vi "CAN Control Timming.vi"() -> ()   [LabVIEW 2010]
uses:
  <vilib>/Platform/storage/lvStorage.llb/xStorage/Open Data Storage/Open Data Storage.xnode
  <vilib>/Platform/storage/lvStorage.llb/_openFunction.ctl
  <vilib>/Platform/storage/lvStorage.llb/xStorage/Set Properties/Set Properties.xnode
  <vilib>/Platform/storage/lvStorage.llb/xStorage/Write Data/Write Data.xnode
  <vilib>/Platform/storage/Storage.llb/usiOverwriteOptions.ctl
  <vilib>/Platform/storage/Storage.llb/usiSequenceRepresentation.ctl
  <vilib>/Platform/storage/lvStorage.llb/xStorage/Close Data Storage/Close Data Storage.xnode
  <instrlib>/Tektronix DPO MSO 2000 4000 Series/Public/Data/Read (Single Waveform).vi
  <instrlib>/Tektronix DPO MSO 2000 4000 Series/Public/Data/Read (Multiple Waveforms).vi
  <vilib>/Platform/storage/lvStorage.llb/_openStorageWithRootAutoDetect.vi
  <vilib>/Platform/storage/lvStorage.llb/xStorage/xStorageSupp/ErrorOut.vi
  <vilib>/Platform/storage/Storage.llb/__savePropString.vi
  <vilib>/Platform/storage/Storage.llb/__savePropTime.vi
  <vilib>/Platform/storage/Storage.llb/_createExplicitChildObject.vi
  <vilib>/Platform/storage/lvStorage.llb/_prepDDT.vi
  <vilib>/Platform/storage/lvStorage.llb/_getChannelNameFromDDT.vi
  <vilib>/Platform/storage/lvStorage.llb/_saveDDT.vi
  <vilib>/Platform/storage/Storage.llb/Get Object Info.vi
  <vilib>/Platform/storage/Storage.llb/__closeStorageFromObject.vi
  <instrlib>/Tektronix DPO MSO 2000 4000 Series/Tektronix DPO MSO 2000 4000 Series.lvlib
panel:
  out "error out":errorcluster
  in  "Error Range":dbl min=0.0 max=5.0 step=0.1 format="%#.3g"
  in  "DPO-4034 IP Adress":string
  in  "Port":u16(ring) items=["AMB 1", "AMB 2", "AMB 3", "AMB 4", "AMB 5", "AMB 18"]
  in  "ABM-S/N":string
  in  "Assembled by":string="Alexis Ibarra"
  in  "Tab Control":enum32{"Diferential"}(tab)
  out "TIMB":waveform(dbl)(graph)
  out "CAN Diferential":waveform(dbl)(graph)
  in  "Maximum Time (10000ms)":u32=20000
  in  "Channel B (1: Channel 2)":u16(ring)=1 items=["Channel 1", "Channel 2", "Channel 3", "Channel 4", "Math", "Reference 1", "Reference 2", "Reference 3", "Reference 4"]
  in  "Channel A (0: Channel 1)":u16(ring) items=["Channel 1", "Channel 2", "Channel 3", "Channel 4", "Math", "Reference 1", "Reference 2", "Reference 3", "Reference 4"]
  out "UP":dbl
  out "DOWN":dbl
  out "?":bool
  out "?":bool
  out "STATUS":string
  out "Delay":dbl format="%^#_6g"
  out "average":dbl
  out "CAN+TIMB":waveform(dbl)[](graph)
  # "TCPIP0::10.195.18.178::inst0::INSTR"
  # "Actually ip address\n10.195.18.178"
  # "%"
  # "Error Limit"
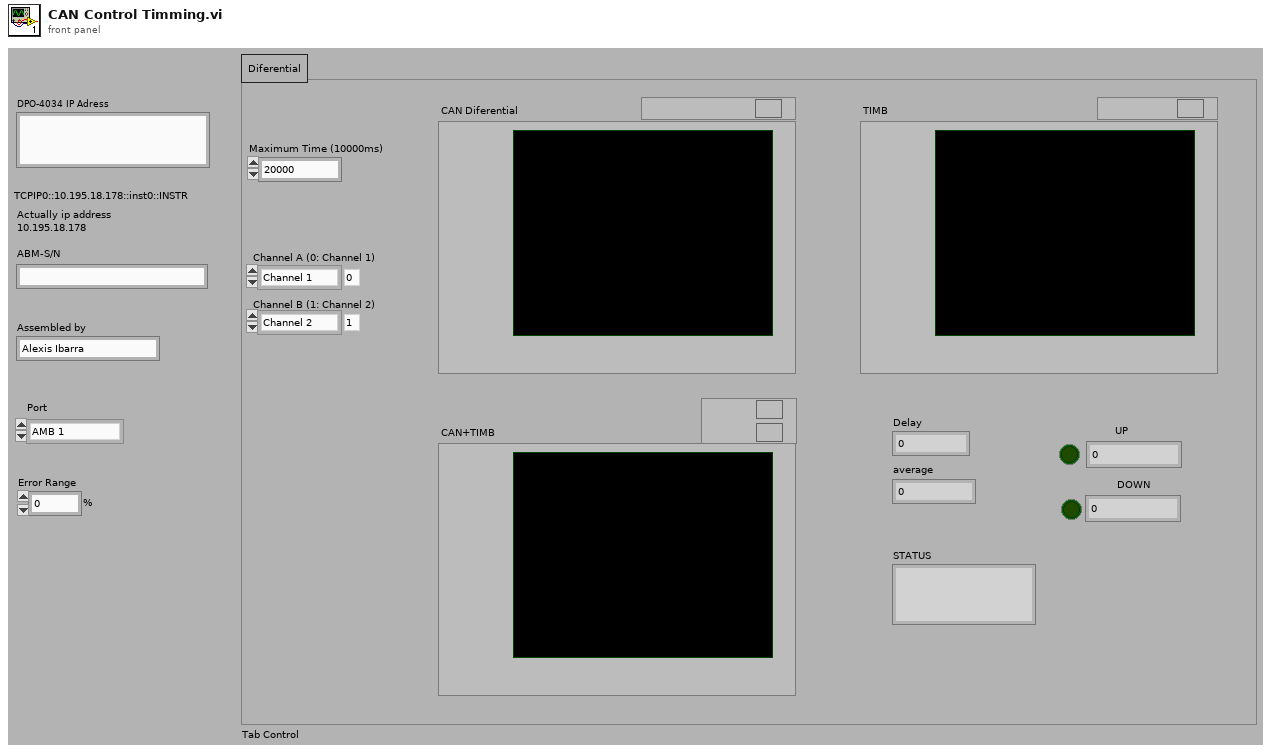
[diagram p1: front panel]
types:
  T1 = enum16{"UPDATE", "READ", "QUERY", "CREATE CHILD", "CREATE", "CONNECT", "DISCONNECT"}
  T2 = typedef "usiOverwriteOptions.ctl" = enum16{"Append values", "Replace values at index", "Replace all values", "Append if timeline aligns"}
  T3 = typedef "usiSequenceRepresentation.ctl" = enum16{"explicit", "implicit"}
  T4 = typedef "_openFunction.ctl" = enum16{"open", "open or create", "create or replace", "create", "open (read only)"}
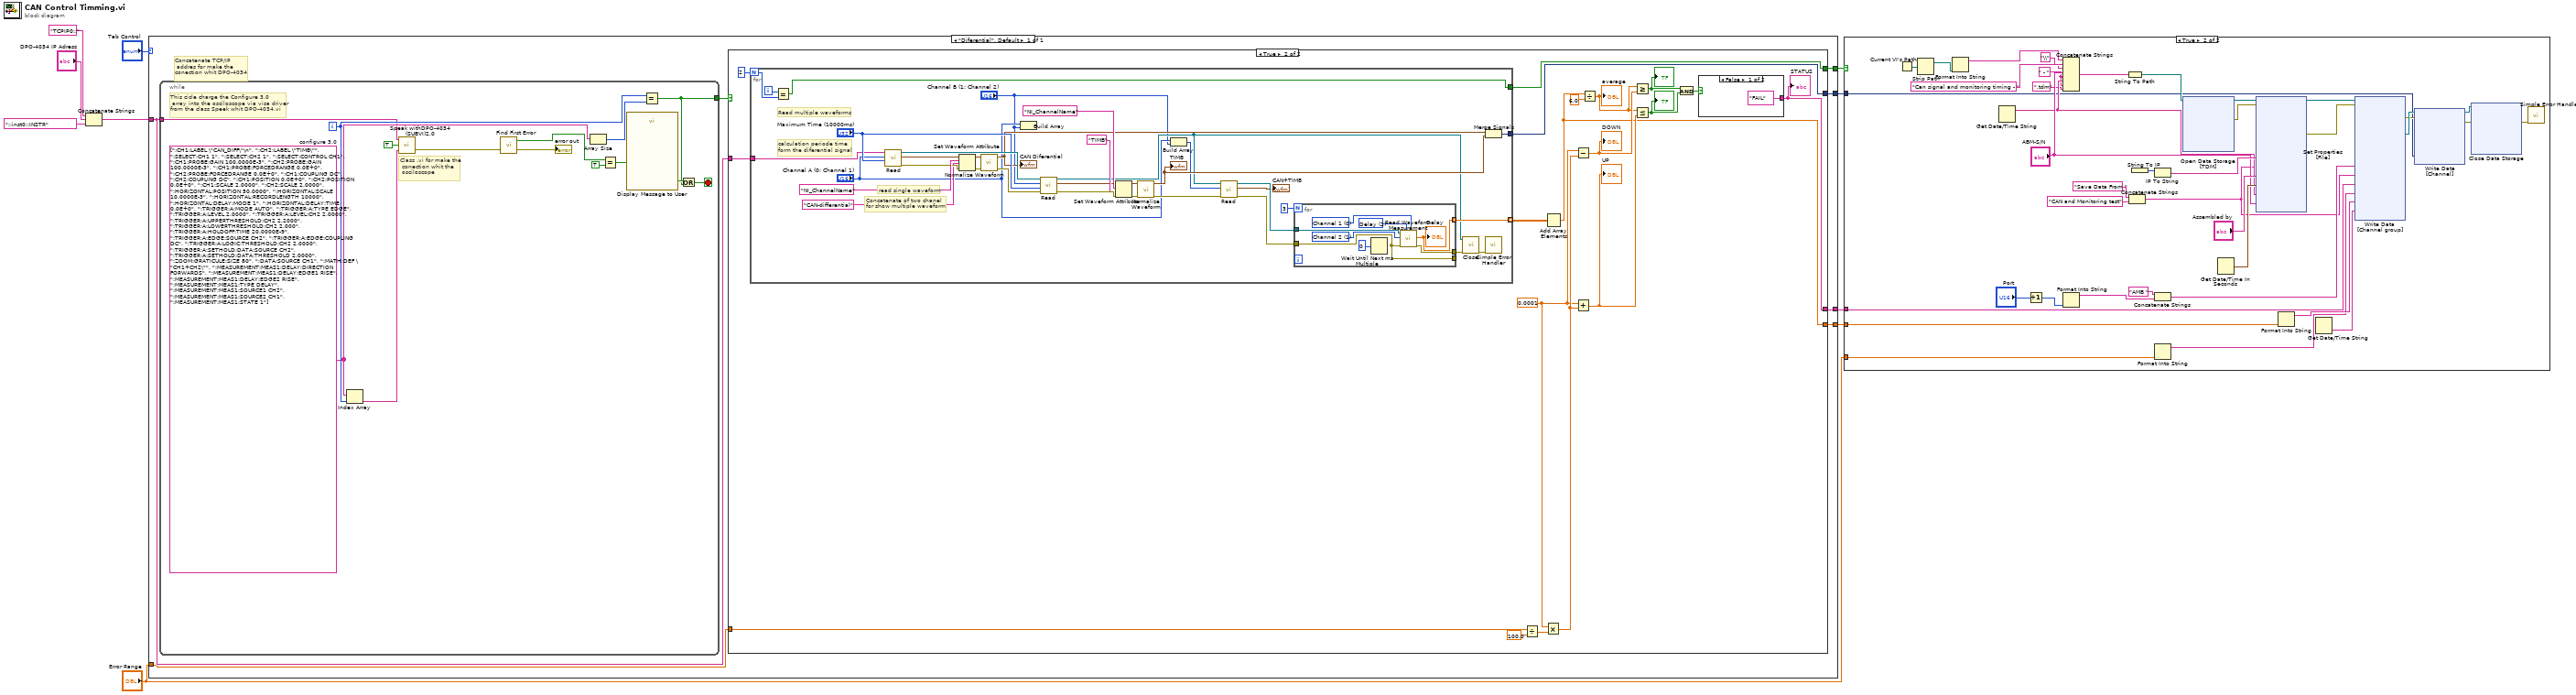
[diagram p0: block diagram]
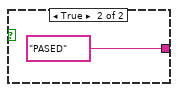
[diagram p4: hidden frame]
diagram:
  n1 = Concatenate Strings("TCPIP0::", "DPO-4034 IP Adress", "::inst0::INSTR") -> (w4:string)
  n2 = case shown="\"Diferential\", Default" "Tab Control" {
    tunnel: [w16] -> w9
    tunnel: [w15] -> w8
    tunnel: w4 -> [w14]
    tunnel: [w13] -> w3
    tunnel: "Error Range" -> [w12]
    tunnel: [w11] -> w1
    frame "Diferential", Default {
      # "Concatenate TCP/IP\n addres for make the \nconection whit DPO-4034"
      n3 = while {
        tunnel: w14 -> [w84]
        tunnel: [w81] -> w17
        i -> [w93]
        stop <- w82 stop-if-true
        w88 = string[] [":CH1:LABEL \"CAN_DIFF\"\n", ":CH2:LABEL \"TIMB\"", ":SELECT:CH1 1", ":SELECT:CH2 1", ":SELECT:CONTROL CH1", ":CH1:PROBE:GAIN 100.0000E-3", ":CH2:PROBE:GAIN 100.0000E-3", ":CH1:PROBE:FORCEDRANGE 0.0E+0", ":CH2:PROBE:FORCEDRANGE 0.0E+0", ":CH1:COUPLING DC", ":CH2:COUPLING DC", ":CH1:POSITION 0.0E+0", ":CH2:POSITION 0.0E+0", ":CH1:SCALE 2.0000", ":CH2:SCALE 2.0000", ":HORIZONTAL:POSITION 50.0000", ":HORIZONTAL:SCALE 10.0000E-3", ":HORIZONTAL:RECORDLENGTH 10000", ":HORIZONTAL:DELAY:MODE 1", ":HORIZONTAL:DELAY:TIME 0.0E+0", ":TRIGGER:A:MODE AUTO", ":TRIGGER:A:TYPE EDGE", ":TRIGGER:A:LEVEL 2.0000", ":TRIGGER:A:LEVEL:CH2 2.0000", ":TRIGGER:A:UPPERTHRESHOLD:CH2 2.2000", ":TRIGGER:A:LOWERTHRESHOLD:CH2 2.000", ":TRIGGER:A:HOLDOFF:TIME 20.0000E-9", ":TRIGGER:A:EDGE:SOURCE CH2", ":TRIGGER:A:EDGE:COUPLING DC", ":TRIGGER:A:LOGIC:THRESHOLD:CH2 2.0000", ":TRIGGER:A:SETHOLD:DATA:SOURCE CH2", ":TRIGGER:A:SETHOLD:DATA:THRESHOLD 2.0000", ":ZOOM:GRATICULE:SIZE 80", ":DATA:SOURCE CH1", ":MATH:DEF \"CH1+CH2\"", ":MEASUREMENT:MEAS1:DELAY:DIRECTION FORWARDS", ":MEASUREMENT:MEAS1:DELAY:EDGE1 RISE", ":MEASUREMENT:MEAS1:DELAY:EDGE2 RISE", ":MEASUREMENT:MEAS1:TYPE DELAY", ":MEASUREMENT:MEAS1:SOURCE1 CH2", ":MEASUREMENT:MEAS1:SOURCE2 CH1", ":MEASUREMENT:MEAS1:STATE 1"]  # configure 3.0
        # "Class .vi for make the\n conection whit the\n osciloscope"
        # "This cicle charge the Configure 3.0\n array into the osciloscope via visa driver \nfrom the class Speek whit DPO-4034.vi"
        n4 = Index Array "Index Array"(array=w88, index=w93) -> (element=w94:string)
        n5 = call "Speak withDPO-4034 (SUBVI)2.0.vi"("Send Command"=w94, "Send:  TRUE\nRecive: FALSE"=TRUE, "VISA Resource Name"=w84) -> ("error out"=w90:errorcluster)  [unwired: 1 out]
        n6 = call <vilib>:"Find First Error.vi"("error in (no error)"=w90) -> ("error out"=→"error out":errorcluster, "error?"=w85:bool)  [unwired: 3 in]
        n7 = Array Size(array=w88) -> (size(s)=w92:i32)
        n8 = Equal?(x=w85, y=TRUE) -> (x = y?=w87:bool)
        n9 = call "Display Message to User"("Enable"=w87) -> ("OK"=w83:bool)  [unwired: 9 in, 1 out]
        n10 = Equal?(x=w93, y=w92) -> (x = y?=w81:bool)
        n11 = Or(x=w83, y=w81) -> (x .or. y?=w82:bool)
      }
      n12 = case shown="True" w17 {
        tunnel: w14 -> [_ w36]
        tunnel: [_ w35] -> w16
        tunnel: [_ w34] -> w15
        tunnel: [_ w20] -> w13
        tunnel: w12 -> [_ w27]
        tunnel: [_ w23] -> w11
        frame False {
        }
        frame True {
          w30 = 0.0001 ("x")
          n13 = for {
            N: 2 -> [w47]
            tunnel: w36 -> [w51]
            tunnel: [w52] -> w35
            tunnel: [w46] -> w34
            tunnel: [w45] -> w18 mode=indexing
            i -> [w48]
            # "read single waveform"
            # "Concatenate of two chanel \nfor show multiple waveform"
            # "calculation periode time\nform the diferential signal"
            # "Read multiple waveforms"
            n14 = Equal?(x=w48, y=w47) -> (x = y?=w46:bool)
            n15 = call-poly <instrlib>:"Read.vi"("Maximum Time (10000ms)"="Maximum Time (10000ms)", "Channel (0: Channel 1)"="Channel A (0: Channel 1)", "VISA resource name"=w51) -> ("error out"=w67:errorcluster, "Waveform Graph"=w56:waveform(dbl), "VISA resource name out"=w69:refnum<visa-resource-name>)  [unwired: 6 in]
            n16 = Set Waveform Attribute(4:w67, 5:"CAN-differential" ("name"), 6:"NI_ChannelName" ("name"), 7:w56) -> (0:w59:errorcluster, 3:w61:waveform(dbl))  [unwired: 1 out]
            n17 = call <vilib>:"Normalize Waveform.vi"("error in (no error)"=w59, "waveform in"=w61) -> ("error out"=w58:errorcluster, "normalized waveform"=w54:waveform(dbl))  [unwired: 6 in, 2 out]
            "CAN Diferential" <- w54
            n18 = Build Array("Channel A (0: Channel 1)", "Channel B (1: Channel 2)") -> ()  [unwired: 1 out]
            n19 = call-poly <instrlib>:"Read.vi"("error in (no error)"=w58, "Maximum Time (10000ms)"="Maximum Time (10000ms)", "Channel (0: Channel 1)"="Channel B (1: Channel 2)", "VISA resource name"=w69) -> ("error out"=w64:errorcluster, "Waveform Graph"=w55:waveform(dbl), "VISA resource name out"=w42:refnum<visa-resource-name>)  [unwired: 5 in]
            n20 = Set Waveform Attribute(4:w64, 5:"TIMB" ("name"), 6:"NI_ChannelName" ("name"), 7:w55) -> (0:w57:errorcluster, 3:w60:waveform(dbl))  [unwired: 1 out]
            n21 = call <vilib>:"Normalize Waveform.vi"("error in (no error)"=w57, "waveform in"=w60) -> ("error out"=w44:errorcluster, "normalized waveform"=w53:waveform(dbl))  [unwired: 6 in, 2 out]
            "TIMB" <- w53
            n22 = Build Array("Channel A (0: Channel 1)", "Channel B (1: Channel 2)") -> (w38:u16[])
            n23 = call-poly <instrlib>:"Read.vi"("error in (no error)"=w44, "Channels"=w38, "VISA resource name"=w42) -> ("error out"=w43:errorcluster, "Waveform Data"=→"CAN+TIMB":waveform(dbl)[], "VISA resource name out"=w41:refnum<visa-resource-name>)  [unwired: 6 in]
            n24 = for {
              N: 3 -> [_]
              tunnel: w41 -> [w78]
              tunnel: [w75] -> _
              tunnel: [w76] -> w50
              tunnel: w43 -> [w75]
              tunnel: [w73] -> w45 mode=indexing
              w71 = u16 0 items=["Channel 1", "Channel 2", "Channel 3", "Channel 4", "MATH", "Reference 1", "Reference 2", "Reference 3", "Reference 4"] ("Destination Channel (1: Channel 2)")
              w72 = u16 1 items=["Channel 1", "Channel 2", "Channel 3", "Channel 4", "MATH", "Reference 1", "Reference 2", "Reference 3", "Reference 4"] ("Channel (0: Channel 1)")
              w74 = 2 items=["Period", "Frequency", "Delay", "Rise Time", "Fall Time", "Positive Duty Cycle", "Negative Duty Cycle", "Positive Pulse Width", "Negative Pulse Width", "Burst Width", "Phase", "Positive Overshoot", "Negative Overshoot", "Vpp", "Amplitude", "Voltage High", "Voltage Low", "Voltage Max", "Voltage Min", "Voltage Mean", "Voltage Mean (cycle)", "Voltage RMS", "Voltage RMS (cycle)", "Area", "Cycle Area", "Positive Edge Count", "Negative Edge Count", "Positive Pulse Count", "Negative Pulse Count"] ("Measurement Function (0: Period)")
              n25 = Wait Until Next ms Multiple(millisecond multiple=u32 0) -> ()  [unwired: 1 out]
              n26 = call <instrlib>:"Read Waveform Measurement.vi"("Destination Channel (1: Channel 2)"=w71, "Measurement Function (0: Period)"=w74, "error in (no error)"=w75, "Channel (0: Channel 1)"=w72, "VISA resource name"=w78) -> ("error out"=w76:errorcluster, "Measurement Value"=w73:dbl)  [unwired: 4 in, 1 out]
              "Delay" <- w73
            }
            n27 = call <instrlib>:"Close.vi"("error in (no error)"=w50, "VISA resource name"=w42) -> ("error out"=w70:errorcluster)  [unwired: 9 in]
            n28 = Merge Signals(w54, w53) -> (w52:dynamicdata)
            n29 = call <vilib>:"Simple Error Handler.vi"("error in (no error)"=w70) -> ()  [unwired: 4 in, 5 out]
          }
          n30 = Divide(x=w27, y=100.0) -> (x/y=w29:dbl)
          n31 = Add Array Elements(numeric array=w18) -> (sum=w20:dbl)
          n32 = Multiply(x=w30, y=w29) -> (x*y=w31:dbl)
          n33 = Subtract(x=w30, y=w31) -> (x-y=w33:dbl)
          "DOWN" <- w33
          n34 = Add(x=w30, y=w31) -> (x+y=w32:dbl)
          "UP" <- w32
          n35 = Divide(x=w20, y=6.0) -> (x/y=w19:dbl)
          "average" <- w19
          n36 = Greater Or Equal?(x=w19, y=w33) -> (x >= y?=w26:bool)
          "?" <- w26
          n37 = Less Or Equal?(x=w19, y=w32) -> (x <= y?=w25:bool)
          "?" <- w25
          n38 = And(x=w26, y=w25) -> (x .and. y?=w24:bool)
          n39 = case shown="False" w24 {
            tunnel: ["FAIL" "PASED"] -> w23
            frame False {
            }
            frame True {
            }
          }
          "STATUS" <- w23
        }
      }
    }
  }
  n40 = case shown="True" w8 {
    tunnel: w9 -> [_ w101]
    tunnel: w3 -> [_ w100]
    tunnel: "Error Range" -> [_ w98]
    tunnel: w1 -> [_ w96]
    frame False {
    }
    frame True {
      w113 = " - " ("string")
      n41 = Current VI's Path() -> (path=w127:path)
      n42 = Strip Path(path=w127) -> (stripped path=w128:path)  [unwired: 1 out]
      n43 = Format Into String "Format Into String"(w128) -> (resulting string=w126:string)  [unwired: 3 in, 1 out]
      n44 = Get Date/Time String() -> (date string=w114:string)  [unwired: 3 in, 1 out]
      n45 = Increment(x="Port") -> (x+1=w102:u16)
      n46 = Concatenate Strings "Concatenate Strings"(w126, "\\", "Can signal and monitoring timing - " ("string"), "ABM-S/N", w113, w114, w113, ".tdm") -> (w130:string)
      n47 = Format Into String "Format Into String"(w102) -> (resulting string=w110:string)  [unwired: 3 in, 1 out]
      n48 = String To Path(string=w130) -> (path=w131:path)
      n49 = Concatenate Strings "Concatenate Strings"("Save Data From ", "CAN and Monitoring test") -> (w104:string)
      n50 = String To IP() -> (0:w120:u32)  [unwired: 1 in]
      n51 = IP To String(2:w120) -> (0:w121:string)  [unwired: 1 in]
      n52 = Concatenate Strings "Concatenate Strings"("AMB ", w110) -> (w107:string)
      n53 = Format Into String "Format Into String"(w98) -> (resulting string=w97:string)  [unwired: 3 in, 1 out]
      n54 = xnode "Open Data Storage\n[TDM]"("file path"=w131) -> ("storage refnum (file)"=w124:refnum<k20>, "error out"=w111:errorcluster)  [unwired: 4 in, 1 out]
      n55 = Get Date/Time In Seconds() -> (seconds since 1Jan1904=w125:timestamp)
      n56 = xnode "Set Properties\n[File]"("Name"=w121, "Description"=w104, "Author"="Assembled by", "Time stamp"=w125, "Date"=w114, "ABM_SerialNumber"="ABM-S/N", "storage refnum (file)"=w124, "error in"=w111) -> ("storage refnum (file) out"=w109:refnum<k20>, "error out"=w108:errorcluster)
      n57 = Format Into String(w100) -> (resulting string=w99:string)  [unwired: 3 in, 1 out]
      n58 = Get Date/Time String() -> (time string=w95:string)  [unwired: 3 in, 1 out]
      n59 = xnode "Write Data\n[Channel group]"("Name"=w107, "Description"=w104, "Status"=w96, "Error_Range"=w97, "Periode"=w99, "Date"=w95, "storage refnum (file)"=w109, "error in"=w108) -> ("error out"=w105:errorcluster, "storage refnum (channel group)"=w106:refnum<k20>)  [unwired: 1 out]
      n60 = xnode "Write Data\n[Channel]"("Signal"=w101, "storage refnum (channel group)"=w106, "error in"=w105) -> ("storage refnum (channel group) out"=w118:refnum<k20>, "error out"=w117:errorcluster)  [unwired: 2 in, 1 out]
      n61 = xnode "Close Data Storage\n"("storage refnum (channel group)"=w118, "error in (no error)"=w117) -> ("error out"=w119:errorcluster)  [unwired: 1 out]
      n62 = call <vilib>:"Simple Error Handler.vi"("error in (no error)"=w119) -> ()  [unwired: 1 in, 8 out]
    }
  }
